vi "LVClass_WavefrontCorrector dtor.vi"(0 "WavefrontCorrector in":refnum<class "WavefrontCorrector.lvclass">, 11 "error in (no error)":errorcluster) -> (4 "WavefrontCorrector out":refnum<class "WavefrontCorrector.lvclass">, 15 "error out":errorcluster)   [LabVIEW 2020, in "WavefrontCorrector.lvclass"]
doc: "WavefrontCorrector destructor.\n\n--------------------------------------------------------------------------------\n\n<B>correctorIn </B> : WavefrontCorrector object.\n<B>correctorOut </B> : WavefrontCorrector object.\n<B>ErrorIn </B> : Error\n<B>ErrorOut </B> : Error\n\n--------------------------------------------------------------------------------"
uses:
  WavefrontCorrector.lvclass
  Wavefront Corrector states - ONE.ctl
  WavefrontCorrector.lvclass/WavefrontCorrector.ctl
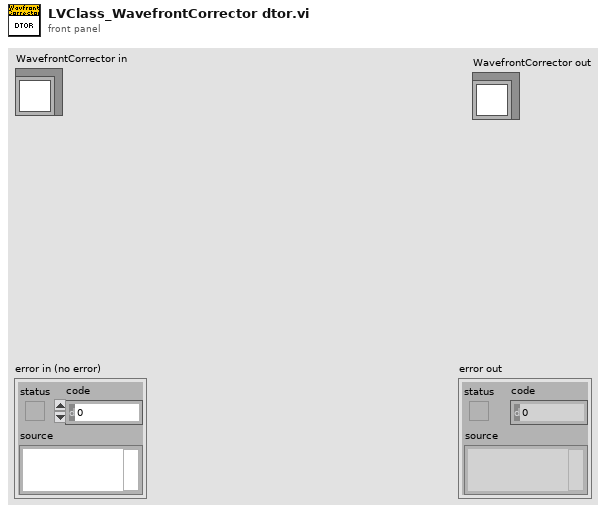
[diagram p1: front panel]
types:
  T1 = typedef "Wavefront Corrector states - ONE.ctl" = cluster{"Max":sgl, "Min":sgl, "Validity":enum16{"valid", "fixed", "invalid"}, "Fixed_Position":sgl}
  T2 = cluster{"Sleep after command apply_ms":i32, "Wavefront Corrector State":T1[]}
  T3 = typedef "Handle creation.ctl" = enum16{"By ctor", "By write function"}
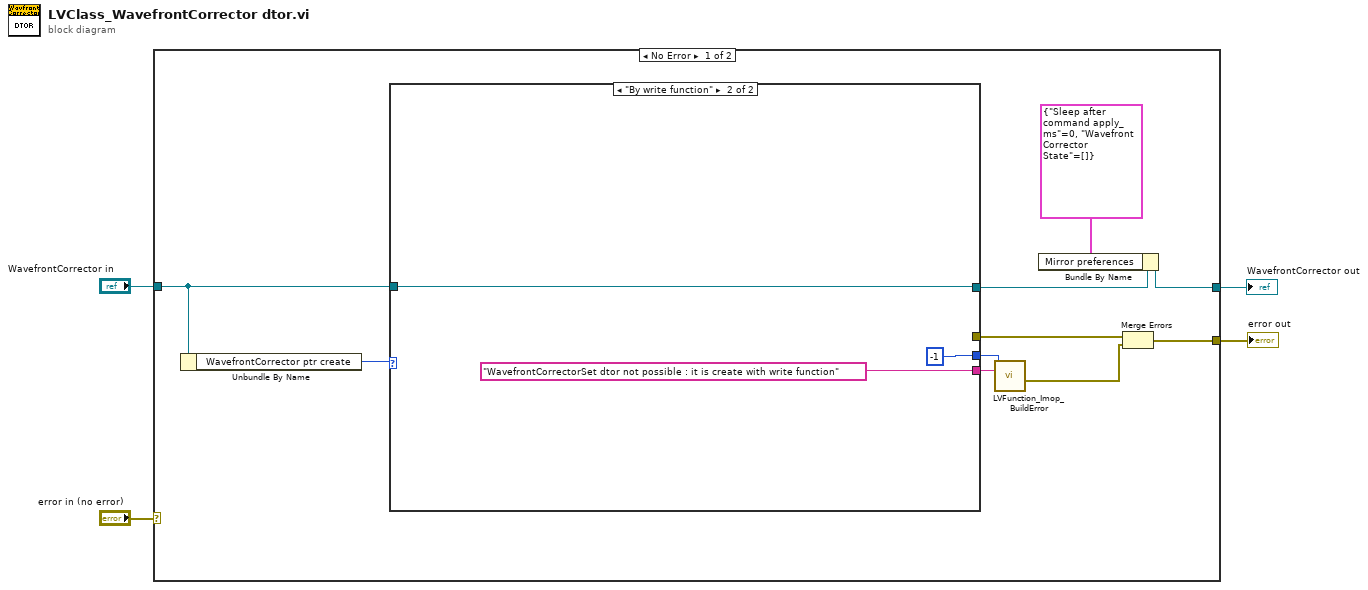
[diagram p0: block diagram]
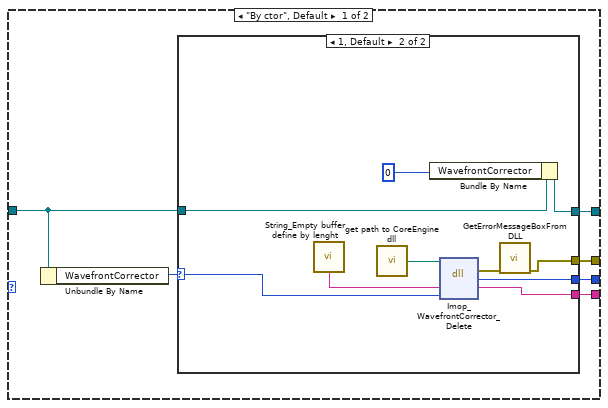
[diagram p2: hidden frame]
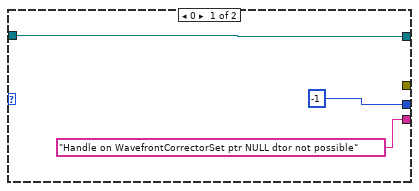
[diagram p3: hidden frame]
diagram:
  n1 = case shown="No Error" "error in (no error)" {
    selector: "error in (no error)" -> [_ w37]
    tunnel: "WavefrontCorrector in" -> [w12 w38]
    tunnel: [w6 w38] -> w1
    tunnel: [w8 w37] -> w2
    frame No Error {
      n2 = Unbundle By Name(w12) -> ("WavefrontCorrector ptr create"=w11:T3)
      n3 = case shown="\"By write function\"" w11 {
        tunnel: [w20 "WavefrontCorrectorSet dtor not possible : it is create with write function" ("message")] -> w14
        tunnel: [w19 -1] -> w13
        tunnel: w12 -> [w17 w34]
        tunnel: [w18 w34] -> w7
        tunnel: [w15 _] -> w10
        frame "By ctor", Default {
          n4 = Unbundle By Name(w17) -> ("WavefrontCorrector"=w16:i32)
          n5 = case shown="1, Default" w16 {
            selector: w16 -> [_ w30]
            tunnel: ["Handle on WavefrontCorrectorSet ptr NULL dtor not possible" ("message") w32] -> w20
            tunnel: [-1 w31] -> w19
            tunnel: w17 -> [w21 w26]
            tunnel: [w21 w25] -> w18
            tunnel: [_ w24] -> w15
            frame 0 {
            }
            frame 1, Default {
              n6 = call "String_Empty buffer define by lenght.vi"() -> ("Empty buffer"=w33:string)  [unwired: 1 in]
              n7 = call "get path to CoreEngine dll.vi"() -> ("path to c_interface_vc100.dll"=w29:path)  [unwired: 12 in, 3 out]
              n8 = Bundle By Name(cluster=w26, "WavefrontCorrector"=u32 0 ("HasoEgine")) -> (w25:refnum<class "WavefrontCorrector.lvclass">)
              n9 = dll-call lib="D:/soft/HASO_v3/SVN_trunk/ImOpCoreEngine4_LV2011/DLLs/c_interface_vc100.dll" fn="Imop_WavefrontCorrector_Delete"(path in=w29, "message"=w33, "WavefrontCorrectionSet"=w30) -> (error out=w28:errorcluster, "return type"=w31:i32, "message"=w32:string)  [unwired: 3 in, 1 out]
              n10 = call "GetErrorMessageBoxFromDLL.vi"("error IN"=w28) -> ("error OUT"=w24:errorcluster)  [unwired: 10 in]
            }
          }
        }
        frame "By write function" {
        }
      }
      n11 = call "LVFunction_Imop_BuildError.vi"("code"=w13, "String to Prepend to source (\"\")"=w14) -> ("error out"=w9:errorcluster)  [unwired: 13 in]
      n12 = Bundle By Name(cluster=w7, "Mirror preferences"=T2 {"Sleep after command apply_ms"=0, "Wavefront Corrector State"=[]}) -> (w6:refnum<class "WavefrontCorrector.lvclass">)
      n13 = Merge Errors(w10, w9) -> (w8:errorcluster)
    }
    frame Error {
    }
  }
  "error out" <- w2
  "WavefrontCorrector out" <- w1
